vi "_FPGA_Aux_ArbWfm.vi"(8 "Cycle in":u64) -> (2 "AuxVoltage":fxp<+/-,16,14>)   [LabVIEW 2018]
uses:
  <vilib>/rvi/Memory/Memory_Emulation/nirvimemoryFastEmulation.vi
  <vilib>/rvi/Memory/Memory_Emulation/nirvimemoryEmulation.vi
  <vilib>/rvi/Emulation/niFpgaEmulationIsFPGAContextNoSignature.vi
  <vilib>/rvi/DataTransferAndStorage/Container/Common/niFpgaContainerGetUniqueNameForEmu.vi
  <vilib>/rvi/Emulation/niFpgaProcessEmulError.vi
  <vilib>/rvi/Emulation/niFpgaSctlEmulationGetInTimedLoop.vi
  <vilib>/rvi/errors/nirviReportUnexpectedCaseInternalError (U32).vi
  <vilib>/rvi/DataTransferAndStorage/Container/XNode/niFpgaContainer.xnode
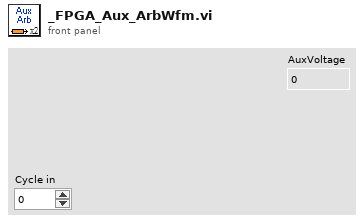
[diagram p1: front panel]
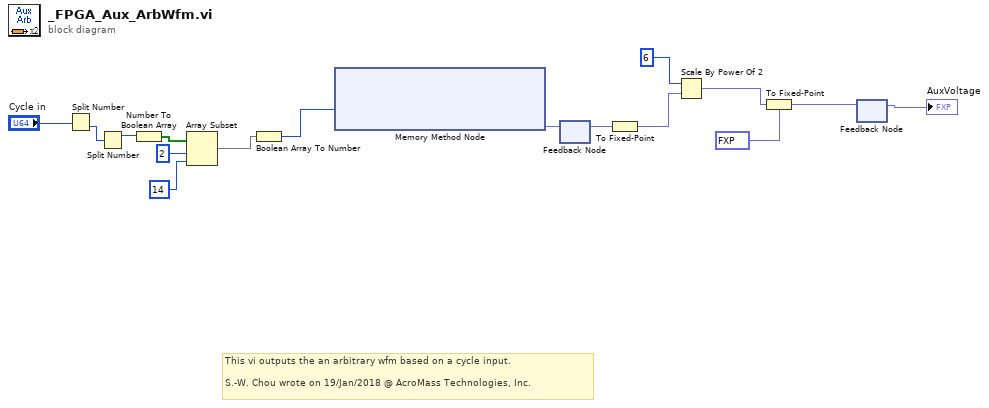
[diagram p0: block diagram]
diagram:
  # "This vi outputs the an arbitrary wfm based on a cycle input.\n\nS.-W. Chou wrote on 19/Jan/2018 @ AcroMass Technologies, Inc."
  n1 = Split Number(x="Cycle in") -> (lo(x)=w12:u32)  [unwired: 1 out]
  n2 = Split Number(x=w12) -> (hi(x)=w11:u16)  [unwired: 1 out]
  n3 = Number To Boolean Array(number=w11) -> (Boolean array=w10:bool[])
  n4 = Array Subset(array=w10, index=2, length=14) -> (w7:bool[])
  n5 = Boolean Array To Number(Boolean array=w7) -> (number=w6:u32)
  n6 = xnode ("Memory Method Node")("Address"=w6) -> ("Data"=w5:fxp<+/-,9,9>)  [unwired: 1 in, 1 out]
  n7 = feedback-in #1(w5) -> ()
  n8 = feedback #1() -> (w2:fxp<+/-,9,9>)  [unwired: 1 in]
  n9 = To Fixed-Point(number=w2) -> (fixed-point=w3:fxp<+/-,15,15>)  [unwired: 1 in]
  n10 = Scale By Power Of 2(n=i16 6, x=w3) -> (x*2^n=w1:fxp<+/-,15,15>)
  n11 = To Fixed-Point(fixed-point type=fxp<+/-,16,14> 8191.0 ("f"), number=w1) -> (fixed-point=w16:fxp<+/-,16,14>)
  n12 = feedback #2() -> (→"AuxVoltage":fxp<+/-,16,14>)  [unwired: 1 in]
  n13 = feedback-in #2(w16) -> ()
